vi "AV3 ANDRÉ.vi"() -> ()   [LabVIEW 2017]
uses:
  <vilib>/LabVIEW Interface for Arduino/Type Defs/Board Type.ctl
  <vilib>/LabVIEW Interface for Arduino/Type Defs/Connection Type.ctl
  <vilib>/LabVIEW Interface for Arduino/Type Defs/Pin Mode.ctl
  <vilib>/LabVIEW Interface for Arduino/LabVIEW Interface for Arduino.lvlib
panel:
  in  "stop":bool
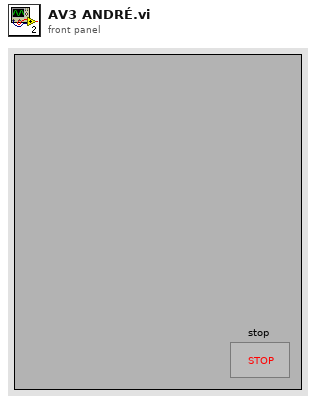
[diagram p1: front panel]
types:
  T1 = typedef "LabVIEW Interface for Arduino.lvlib/Connection Type.ctl" = enum8{"USB / Serial", "XBEE", "BlueSmirf (Bluetooth)"}
  T2 = typedef "LabVIEW Interface for Arduino.lvlib/Board Type.ctl" = enum16{"Uno", "Dimuelanove w/Atmega 328", "Mega 2560"}
  T3 = typedef "LabVIEW Interface for Arduino.lvlib/Arduino Resource.ctl" = cluster{"VISA resource":refnum<visa-resource-name>, "Board Type":T2, "Connection Type":enum8{"USB / Serial"}, "Bytes Per Packet (15)":u8}
  T4 = typedef "LabVIEW Interface for Arduino.lvlib/Pin Mode.ctl" = enum8{"Input", "Output"}
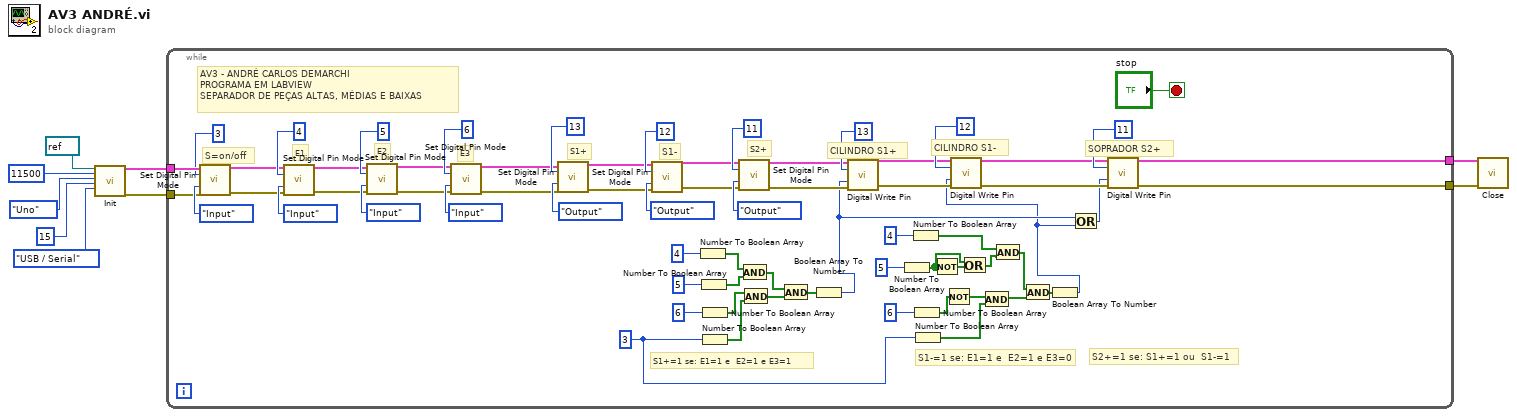
[diagram p0: block diagram]
diagram:
  n1 = call <vilib>:"Init.vi"("VISA resource"=refnum<visa-resource-name> refnum, "Baud Rate (115200)"=u32 11500, "Board Type (Uno)"=Board_Type."Uno", "Bytes Per Packet (15)"=u32 15, "Connection Type (USB/Serial)"=Connection_Type."USB / Serial") -> ("Arduino Resource"=w4:T3, "error out"=w3:errorcluster)  [unwired: 13 in]
  n2 = while {
    tunnel: w4 -> [w53]
    tunnel: w3 -> [w54]
    tunnel: [w31] -> w2
    tunnel: [w30] -> w1
    stop <- "stop" stop-if-true
    w16 = u8 3 ("Value (0)")
    # "S2+=1 se: S1+=1 ou  S1-=1"
    # "S1-=1 se: E1=1 e  E2=1 e E3=0"
    # "AV3 - ANDRÉ CARLOS DEMARCHI\nPROGRAMA EM LABVIEW\nSEPARADOR DE PEÇAS ALTAS, MÉDIAS E BAIXAS"
    # "S1+=1 se: E1=1 e  E2=1 e E3=1"
    # "CILINDRO S1-"
    # "SOPRADOR S2+"
    # "CILINDRO S1+"
    # "S2+"
    # "S1-"
    # "S1+"
    # "E3"
    # "E2"
    # "E1"
    # "S=on/off"
    n3 = call <vilib>:"Set Digital Pin Mode.vi"("Arduino Resource"=w53, "Digital I/O Pin"=u8 3, "Pin Mode (Input)"=Pin_Mode."Input", "error in"=w54) -> ("Arduino Resource"=w38:T3, "error out"=w37:errorcluster)  [unwired: 10 in]
    n4 = call <vilib>:"Set Digital Pin Mode.vi"("Arduino Resource"=w38, "Digital I/O Pin"=u8 4, "Pin Mode (Input)"=Pin_Mode."Input", "error in"=w37) -> ("Arduino Resource"=w52:T3, "error out"=w49:errorcluster)  [unwired: 10 in]
    n5 = call <vilib>:"Set Digital Pin Mode.vi"("Arduino Resource"=w52, "Digital I/O Pin"=u8 5, "Pin Mode (Input)"=Pin_Mode."Input", "error in"=w49) -> ("Arduino Resource"=w51:T3, "error out"=w50:errorcluster)  [unwired: 10 in]
    n6 = call <vilib>:"Set Digital Pin Mode.vi"("Arduino Resource"=w51, "Digital I/O Pin"=u8 6, "Pin Mode (Input)"=Pin_Mode."Input", "error in"=w50) -> ("Arduino Resource"=w36:T3, "error out"=w35:errorcluster)  [unwired: 10 in]
    n7 = call <vilib>:"Set Digital Pin Mode.vi"("Arduino Resource"=w36, "Digital I/O Pin"=u8 13, "Pin Mode (Input)"=Pin_Mode."Output", "error in"=w35) -> ("Arduino Resource"=w47:T3, "error out"=w48:errorcluster)  [unwired: 10 in]
    n8 = call <vilib>:"Set Digital Pin Mode.vi"("Arduino Resource"=w47, "Digital I/O Pin"=u8 12, "Pin Mode (Input)"=Pin_Mode."Output", "error in"=w48) -> ("Arduino Resource"=w46:T3, "error out"=w45:errorcluster)  [unwired: 10 in]
    n9 = Number To Boolean Array(number=u8 4) -> (Boolean array=w61:bool[])
    n10 = Number To Boolean Array(number=u32 5) -> (Boolean array=w60:bool[])
    n11 = Number To Boolean Array(number=u32 6) -> (Boolean array=w21:bool[])
    n12 = Number To Boolean Array(number=w16) -> (Boolean array=w20:bool[])
    n13 = call <vilib>:"Set Digital Pin Mode.vi"("Arduino Resource"=w46, "Digital I/O Pin"=u8 11, "Pin Mode (Input)"=Pin_Mode."Output", "error in"=w45) -> ("Arduino Resource"=w34:T3, "error out"=w33:errorcluster)  [unwired: 10 in]
    n14 = And(x=w61, y=w60) -> (x .and. y?=w59:bool[])
    n15 = And(x=w21, y=w20) -> (x .and. y?=w22:bool[])
    n16 = And(x=w59, y=w22) -> (x .and. y?=w58:bool[])
    n17 = Boolean Array To Number(Boolean array=w58) -> (number=w15:u32)
    n18 = call <vilib>:"Digital Write Pin.vi"("Arduino Resource"=w34, "Digital I/O Pin (0)"=u8 13, "Value (0)"=w15, "error in"=w33) -> ("Arduino Resource"=w43:T3, "error out"=w44:errorcluster)  [unwired: 10 in]
    n19 = Number To Boolean Array(number=u32 5) -> (Boolean array=w10:bool[])
    n20 = Number To Boolean Array(number=u8 4) -> (Boolean array=w28:bool[])
    n21 = Number To Boolean Array(number=u32 6) -> (Boolean array=w24:bool[])
    n22 = Number To Boolean Array(number=w16) -> (Boolean array=w17:bool[])
    n23 = Not(x=w10) -> (.not. x?=w12:bool[])
    n24 = Not(x=w24) -> (.not. x?=w18:bool[])
    n25 = Or(x=w10, y=w12) -> (x .or. y?=w11:bool[])
    n26 = And(x=w18, y=w17) -> (x .and. y?=w19:bool[])
    n27 = And(x=w28, y=w11) -> (x .and. y?=w27:bool[])
    n28 = And(x=w27, y=w19) -> (x .and. y?=w26:bool[])
    n29 = Boolean Array To Number(Boolean array=w26) -> (number=w14:u32)
    n30 = call <vilib>:"Digital Write Pin.vi"("Arduino Resource"=w43, "Digital I/O Pin (0)"=u8 12, "Value (0)"=w14, "error in"=w44) -> ("Arduino Resource"=w40:T3, "error out"=w39:errorcluster)  [unwired: 10 in]
    n31 = Or(x=w15, y=w14) -> (x .or. y?=w13:u32)
    n32 = call <vilib>:"Digital Write Pin.vi"("Arduino Resource"=w40, "Digital I/O Pin (0)"=u8 11, "Value (0)"=w13, "error in"=w39) -> ("Arduino Resource"=w31:T3, "error out"=w30:errorcluster)  [unwired: 10 in]
  }
  n33 = call <vilib>:"Close.vi"("Arduino Resource"=w2, "error in"=w1) -> ()  [unwired: 13 in, 1 out]
